vi "get_stringGenerator.vi"(8 "error in (no error)":errorcluster, 11 "StimulatorAK101022TCP in":refnum<class "StimulatorAK101022TCP.lvclass">) -> (0 "error out":errorcluster, 2 "stringGenerator":refnum<class "GenericStringGenerator.lvclass">, 3 "StimulatorAK101022TCP out":refnum<class "StimulatorAK101022TCP.lvclass">)   [LabVIEW 2010, in "StimulatorAK101022TCP.lvclass"]
uses:
  StimulatorAK101022TCP.lvclass
  StringGenerator/GenericStringGenerator/GenericStringGenerator/GenericStringGenerator.lvclass
  StimulatorAK101022TCP.lvclass/StimulatorAK101022TCP.ctl
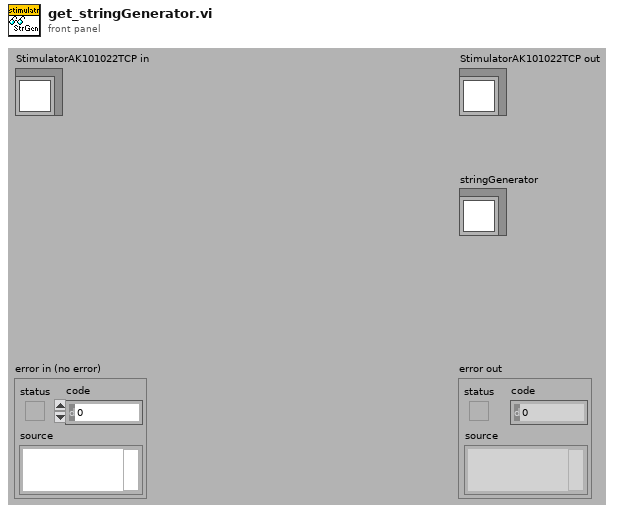
[diagram p1: front panel]
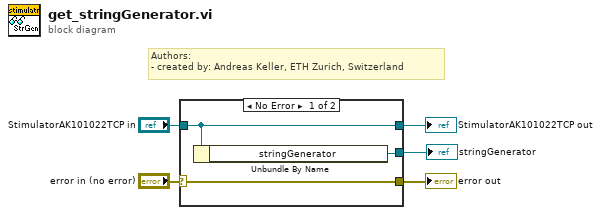
[diagram p0: block diagram]
diagram:
  # "Authors: \n- created by: Andreas Keller, ETH Zurich, Switzerland"
  n1 = case shown="No Error" "error in (no error)" {
    selector: "error in (no error)" -> [w8 w10]
    tunnel: [w8 w10] -> w4
    tunnel: [w7 w9] -> w2
    tunnel: "StimulatorAK101022TCP in" -> [w7 w9]
    tunnel: [w6 _] -> w1
    frame No Error {
      n2 = Unbundle By Name(w7) -> ("stringGenerator"=w6:refnum<class "GenericStringGenerator.lvclass">)
    }
    frame Error {
    }
  }
  "error out" <- w4
  "StimulatorAK101022TCP out" <- w2
  "stringGenerator" <- w1
